vi "ControlPanel_Basic_AC.vi"() -> ()   [LabVIEW 2017]
uses:
  Cornerstone SubVI's/monochromatorConnect.vi
  Cornerstone SubVI's/monochromatorInitialize.vi
  Cornerstone SubVI's/monochromatorDisconnect.vi
  Cornerstone SubVI's/monochromatorCommandSetGrating.vi
  Cornerstone SubVI's/monochromatorCommandGetGrating.vi
  Cornerstone SubVI's/monochromatorCommandSetWavelength.vi
  Cornerstone SubVI's/monochromatorCommandSetShutter.vi
  Cornerstone SubVI's/monochromatorCommandGetShutter.vi
  Cornerstone SubVI's/monochromatorCommandSetSteps.vi
  Cornerstone SubVI's/monochromatorCommandGetWavelength.vi
  C:/Project Work/icl-optical-software-rewrite/Third Party Drivers/Monochromator/Newport - Oriel Instruments/Cornerstone Series Monochromator - API/Cornerstone DLL/Cornerstone.dll
  Cornerstone DLL/Cornerstone.dll
panel:
  in  "MainScreenCtrlPanel":enum32{"Page 1"}(tab)
  in  "Get G":bool
  in  "btn.Shutter":bool
  in  "btn.FastBackward":bool
  in  "btn.Backward":bool
  in  "btn.FastForward":bool
  in  "btn.Forward":bool
  in  "Wavelength":dbl=555.0 caption="nm" min=0.0 format="%.2f"
  out "grating":string
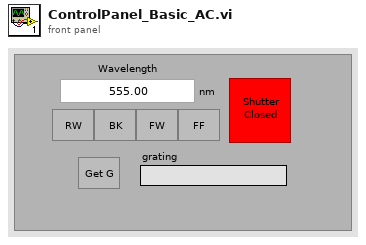
[diagram p1: front panel]
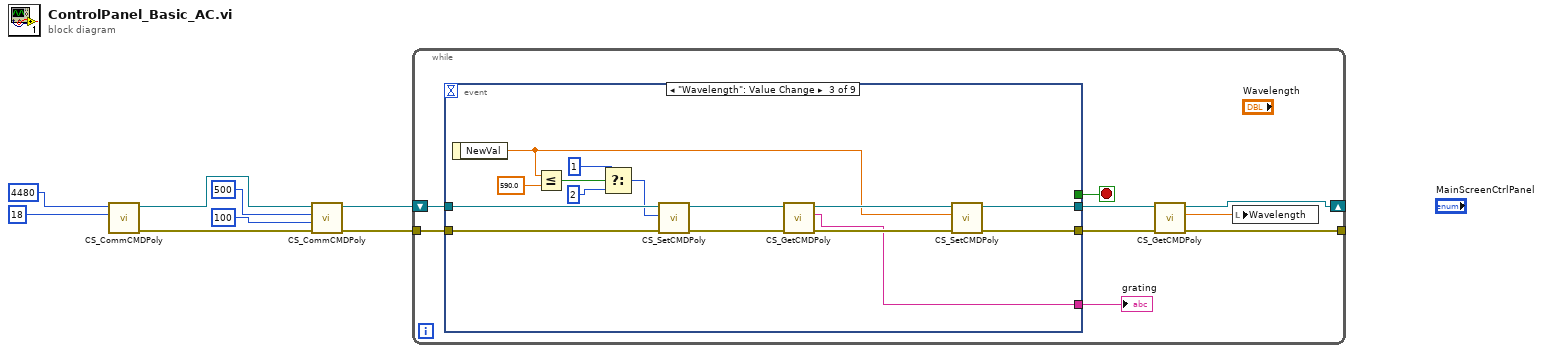
[diagram p0: block diagram]
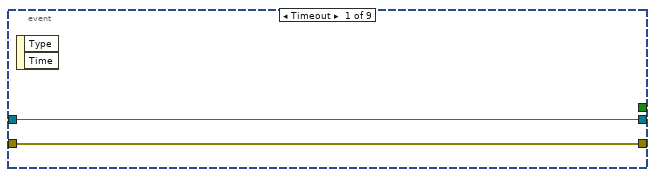
[diagram p2: hidden frame]
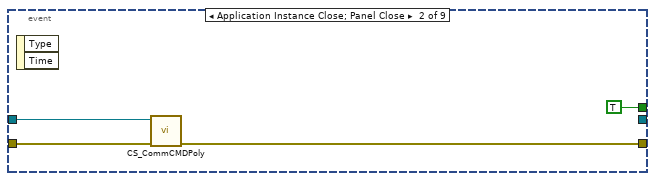
[diagram p3: hidden frame]
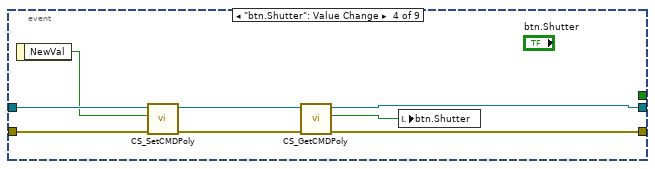
[diagram p4: hidden frame]
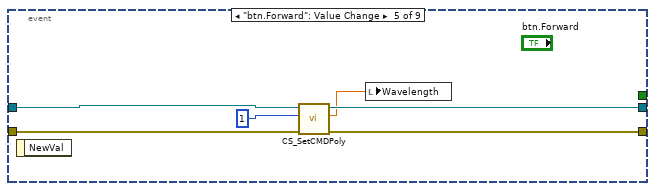
[diagram p5: hidden frame]
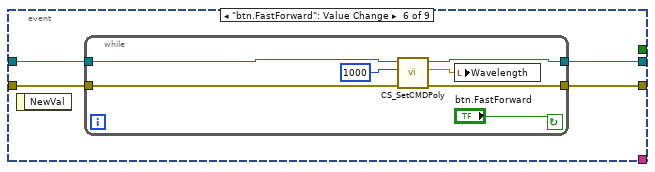
[diagram p6: hidden frame]
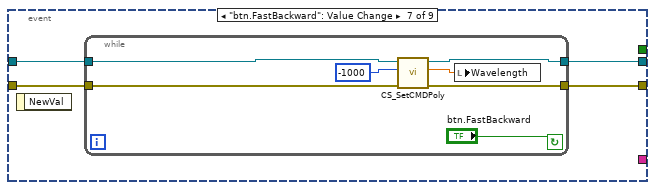
[diagram p7: hidden frame]
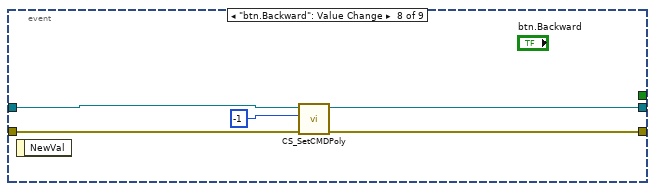
[diagram p8: hidden frame]
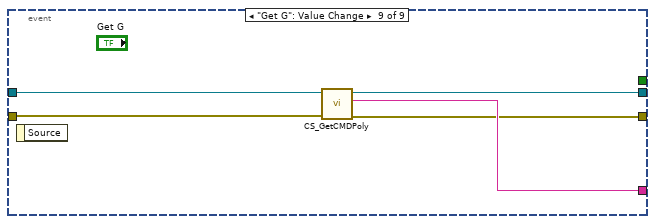
[diagram p9: hidden frame]
diagram:
  n1 = call-poly "CS_CommCMDPoly.vi"("product_id"=18, "vendor_id"=4480) -> ("error out"=w2:errorcluster, "monochromator"=w8:refnum<k24>)  [unwired: 8 in]
  n2 = call-poly "CS_CommCMDPoly.vi"("error in"=w2, "command_wait_time"=100, "dev_timeout"=u32 500, "monochromator"=w8) -> ("error out"=w1:errorcluster, "reference out"=w3:refnum<k24>)  [unwired: 6 in]
  n3 = while {
    tunnel: w1 -> [w15]
    shift-right: [w13] -> _
    shift-left: w3 -> [w16]
    tunnel: [w10] -> _
    stop <- w17 stop-if-true
    n4 = event shown="[2] \"Wavelength\": Value Change" {
      selector: _ -> [_ _ _ _ _ _ _ _ _]
      dyn-events: _ -> [_ _ _ _ _ _ _ _ _]
      timeout: _ -> [_ _ _ _ _ _ _ _ _]
      tunnel: [_ TRUE _ _ _ _ _ _ _] -> w17
      tunnel: w16 -> [w19 w22 w33 w45 w51 w56 w67 w79 w81]
      tunnel: w15 -> [w18 w21 w35 w46 w52 w55 w66 w78 w82]
      tunnel: [w18 w20 w37 w39 w48 w53 w64 w77 w83] -> w11
      tunnel: [w19 _ w38 w42 w49 w54 w65 w76 w80] -> w12
      tunnel: [_ _ w24 _ _ _ _ _ w84] -> w9
      event Timeout {
        n5 = event-data() -> ()  [unwired: 1 in, 2 out]
      }
      event Application Instance Close; Panel Close {
        n6 = event-data() -> ()  [unwired: 1 in, 2 out]
        n7 = call-poly "CS_CommCMDPoly.vi"("error in"=w21, "monochromator"=w22) -> ("error out"=w20:errorcluster)  [unwired: 9 in]
      }
      event "Wavelength": Value Change {
        n8 = event-data() -> ("NewVal"=w30:dbl)  [unwired: 1 in]
        n9 = Less Or Equal?(x=w30, y=590.0) -> (x <= y?=w28:bool)
        n10 = Select(t=1, s=w28, f=2 ("t")) -> (s? t:f=w25:i32)
        n11 = call-poly "CS_SetCMDPoly.vi"("error in"=w35, "grating"=w25, "monochromator"=w33) -> ("error out"=w36:errorcluster, "monochromator"=w31:refnum<k24>)  [unwired: 6 in, 1 out]
        n12 = call-poly "CS_GetCMDPoly.vi"("error in"=w36, "monochromator"=w31) -> ("error out"=w34:errorcluster, "grating"=w24:string, "monochromator"=w32:refnum<k24>)  [unwired: 7 in]
        n13 = call-poly "CS_SetCMDPoly.vi"("error in"=w34, "wavelength"=w30, "monochromator"=w32) -> ("error out"=w37:errorcluster, "monochromator"=w38:refnum<k24>)  [unwired: 6 in, 1 out]
      }
      event "btn.Shutter": Value Change {
        n14 = event-data() -> ("NewVal"=w44:bool)  [unwired: 1 in]
        n15 = call-poly "CS_SetCMDPoly.vi"("error in"=w46, "shutter"=w44, "monochromator"=w45) -> ("error out"=w40:errorcluster, "monochromator"=w43:refnum<k24>)  [unwired: 7 in]
        n16 = call-poly "CS_GetCMDPoly.vi"("error in"=w40, "monochromator"=w43) -> ("error out"=w39:errorcluster, "shutter"=w41:bool, "monochromator"=w42:refnum<k24>)  [unwired: 6 in, 1 out]
        n17 = local write "btn.Shutter"(w41) -> ()
      }
      event "btn.Forward": Value Change {
        n18 = event-data() -> ()  [unwired: 1 in, 1 out]
        n19 = call-poly "CS_SetCMDPoly.vi"("error in"=w52, "step"=1, "monochromator"=w51) -> ("error out"=w48:errorcluster, "wavelength"=w47:dbl, "monochromator"=w49:refnum<k24>)  [unwired: 6 in]
        n20 = local write "Wavelength"(w47) -> ()
      }
      event "btn.FastForward": Value Change {
        n21 = event-data() -> ()  [unwired: 1 in, 1 out]
        n22 = while {
          tunnel: w56 -> [w63]
          tunnel: w55 -> [w62]
          tunnel: [w57] -> w54
          tunnel: [w58] -> w53
          stop <- "btn.FastForward" continue-if-true
          n23 = call-poly "CS_SetCMDPoly.vi"("error in"=w62, "step"=1000, "monochromator"=w63) -> ("error out"=w58:errorcluster, "wavelength"=w59:dbl, "monochromator"=w57:refnum<k24>)  [unwired: 6 in]
          n24 = local write "Wavelength"(w59) -> ()
        }
      }
      event "btn.FastBackward": Value Change {
        n25 = event-data() -> ()  [unwired: 1 in, 1 out]
        n26 = while {
          tunnel: [w69] -> w65
          tunnel: [w70] -> w64
          tunnel: w67 -> [w73]
          tunnel: w66 -> [w72]
          stop <- "btn.FastBackward" continue-if-true
          n27 = call-poly "CS_SetCMDPoly.vi"("error in"=w72, "step"=-1000, "monochromator"=w73) -> ("error out"=w70:errorcluster, "wavelength"=w68:dbl, "monochromator"=w69:refnum<k24>)  [unwired: 6 in]
          n28 = local write "Wavelength"(w68) -> ()
        }
      }
      event "btn.Backward": Value Change {
        n29 = event-data() -> ()  [unwired: 1 in, 1 out]
        n30 = call-poly "CS_SetCMDPoly.vi"("error in"=w78, "step"=-1, "monochromator"=w79) -> ("error out"=w77:errorcluster, "monochromator"=w76:refnum<k24>)  [unwired: 6 in, 1 out]
      }
      event "Get G": Value Change {
        n31 = event-data() -> ()  [unwired: 1 in, 1 out]
        n32 = call-poly "CS_GetCMDPoly.vi"("error in"=w82, "monochromator"=w81) -> ("error out"=w83:errorcluster, "grating"=w84:string, "monochromator"=w80:refnum<k24>)  [unwired: 7 in]
      }
    }
    "grating" <- w9
    n33 = call-poly "CS_GetCMDPoly.vi"("error in"=w11, "monochromator"=w12) -> ("error out"=w10:errorcluster, "wavelength"=w14:dbl, "monochromator"=w13:refnum<k24>)  [unwired: 7 in]
    n34 = local write "Wavelength"(w14) -> ()
  }
